vi "CompareInitConfig(PortConfig).vi"(10 "PortConfig - existing":u32[](array[ring]) items=["FDX_SINGLE", "FDX_REDUNDANT"], 11 "PortConfig - New":T1 {"Port1ConfigIn" items=["FDX_SINGLE", "FDX_REDUNDANT"]; "Port2ConfigIn" items=["FDX_SINGLE", "FDX_REDUNDANT"]; "Port3ConfigIn" items=["FDX_SINGLE", "FDX_REDUNDANT"]; "Port4ConfigIn" items=["FDX_SINGLE", "FDX_REDUNDANT"]}) -> (2 "not equal":bool, 3 "PortConfig - New out":T1 {"Port1ConfigIn" items=["FDX_SINGLE", "FDX_REDUNDANT"]; "Port2ConfigIn" items=["FDX_SINGLE", "FDX_REDUNDANT"]; "Port3ConfigIn" items=["FDX_SINGLE", "FDX_REDUNDANT"]; "Port4ConfigIn" items=["FDX_SINGLE", "FDX_REDUNDANT"]})   [LabVIEW 2020, in "AIM664LV.lvlib"]
uses:
  AIM664LV.lvlib
  _controls/initialize_PortConfig.ctl
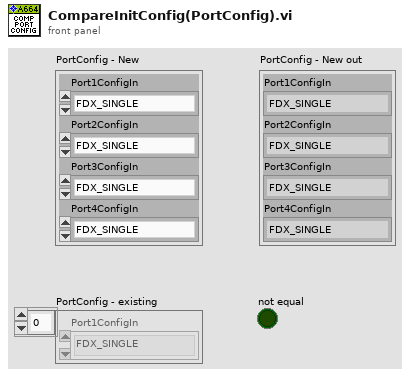
[diagram p1: front panel]
types:
  T1 = typedef "AIM664LV.lvlib/initialize_PortConfig.ctl" = cluster{"Port1ConfigIn":u32, "Port2ConfigIn":u32, "Port3ConfigIn":u32, "Port4ConfigIn":u32}
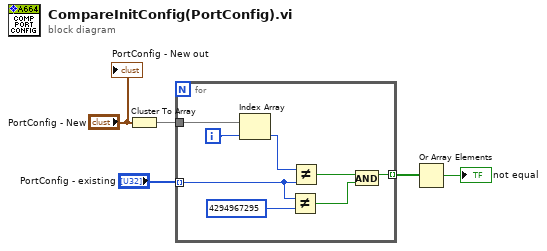
[diagram p0: block diagram]
diagram:
  n1 = Cluster To Array(cluster="PortConfig - New") -> (array=w3:u32[])
  n2 = for {
    tunnel: "PortConfig - existing" -> [w9] mode=indexing
    tunnel: w3 -> [w13]
    tunnel: [w7] -> w2 mode=indexing
    i -> [w12]
    n3 = Index Array(array=w13, index=w12) -> (element=w11:u32)
    n4 = Not Equal?(x=w9, y=u32 4294967295) -> (x != y?=w6:bool)
    n5 = Not Equal?(x=w11, y=w9) -> (x != y?=w10:bool)
    n6 = And(x=w10, y=w6) -> (x .and. y?=w7:bool)
  }
  n7 = Or Array Elements(Boolean array=w2) -> (logical OR=→"not equal":bool)
  "PortConfig - New out" <- "PortConfig - New"
